vi "LabVIEW_PROJECT1.vi"() -> ()   [LabVIEW 2021]
uses:
  <vilib>/Instr/_visa.llb/VISA Configure Serial Port (Instr).vi
panel:
  out "decimal integer string 2":string
  in  "send":bool
  out "decimal integer string":string
  in  "Knob":dbl(knob) scale=0.0..20.0
  in  "COM":refnum<visa-resource-name>
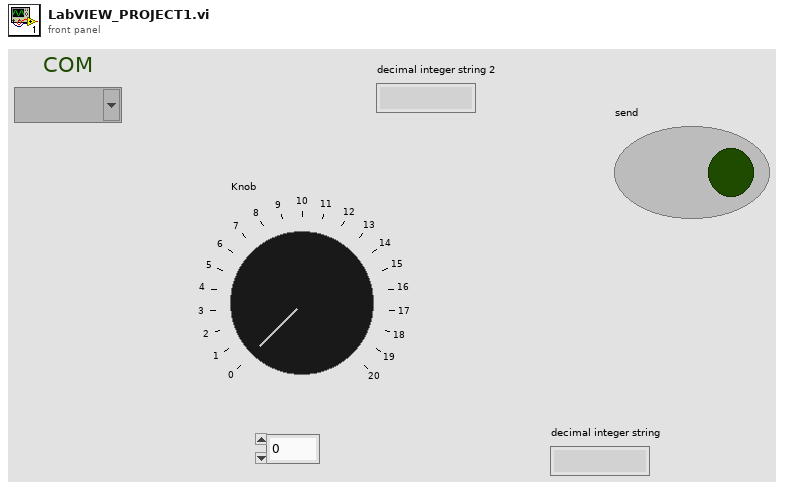
[diagram p1: front panel]
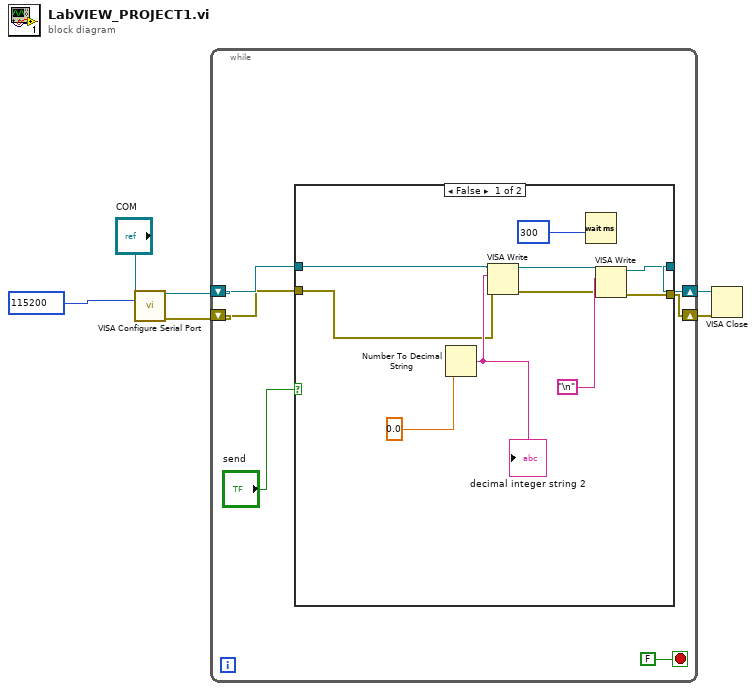
[diagram p0: block diagram]
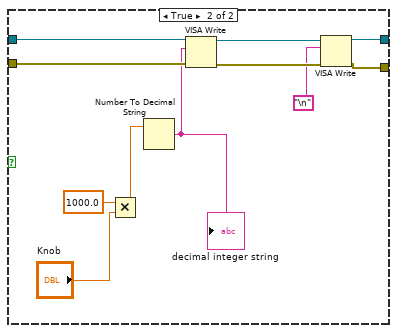
[diagram p2: hidden frame]
diagram:
  n1 = call-poly "VISA Configure Serial Port"("VISA resource name"="COM", "baud rate (9600)"=u32 115200) -> ("VISA resource name out"=w6:refnum<visa-resource-name>, "error out"=w4:errorcluster)  [unwired: 12 in]
  n2 = while {
    shift-right: [w11] -> w5
    shift-left: w6 -> [w12]
    shift-right: [w7] -> w3
    shift-left: w4 -> [w10]
    stop <- FALSE stop-if-true
    n3 = case shown="False" "send" {
      tunnel: w12 -> [w19 w33]
      tunnel: [w17 w31] -> w11
      tunnel: w10 -> [w13 w30]
      tunnel: [w18 w23] -> w7
      frame False {
        n4 = Number To Decimal String(number=0.0 ("x")) -> (decimal integer string=w22:string)  [unwired: 1 in]
        "decimal integer string 2" <- w22
        n5 = VISA Write(VISA resource name=w19, write buffer=w22, error in (no error)=w13) -> (VISA resource name out=w16:refnum<visa-resource-name>, error out=w15:errorcluster)  [unwired: 1 out]
        n6 = Wait (ms)(milliseconds to wait=u32 300) -> ()  [unwired: 1 out]
        n7 = VISA Write(VISA resource name=w16, write buffer="\n", error in (no error)=w15) -> (VISA resource name out=w17:refnum<visa-resource-name>, error out=w18:errorcluster)  [unwired: 1 out]
      }
      frame True {
        n8 = Multiply(x=1000.0, y="Knob") -> (x*y=w24:dbl)
        n9 = Number To Decimal String(number=w24) -> (decimal integer string=w27:string)  [unwired: 1 in]
        "decimal integer string" <- w27
        n10 = VISA Write(VISA resource name=w33, write buffer=w27, error in (no error)=w30) -> (VISA resource name out=w32:refnum<visa-resource-name>, error out=w29:errorcluster)  [unwired: 1 out]
        n11 = VISA Write(VISA resource name=w32, write buffer="\n", error in (no error)=w29) -> (VISA resource name out=w31:refnum<visa-resource-name>, error out=w23:errorcluster)  [unwired: 1 out]
      }
    }
  }
  n12 = VISA Close(VISA resource name=w5, error in (no error)=w3) -> ()  [unwired: 1 out]
